vi "Read S-parameter Magnitude-Phase Pair.vi"(8 "error in (no error)":errorcluster, 10 "S-parameter Type (0: S11)":i32(ring) items=["S11", "S12", "S21", "S22"], 11 "VISA resource name":refnum<visa-resource-name>) -> (0 "error out":errorcluster, 1 "Current Phase":dbl, 2 "Current Magnitude":dbl, 3 "VISA resource name out":refnum<visa-resource-name>)   [LabVIEW 2014, in "Agilent U2000 Series.lvlib"]
doc: "Reads the current magnitude-phase pair values for the specified S-parameter type.\n\nNote: \nThis VI is only applicable for U2040 X-Series."
uses:
  Agilent U2000 Series.lvlib
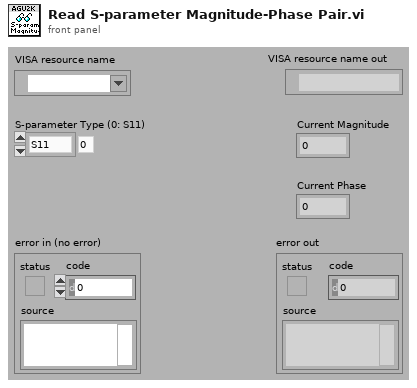
[diagram p1: front panel]
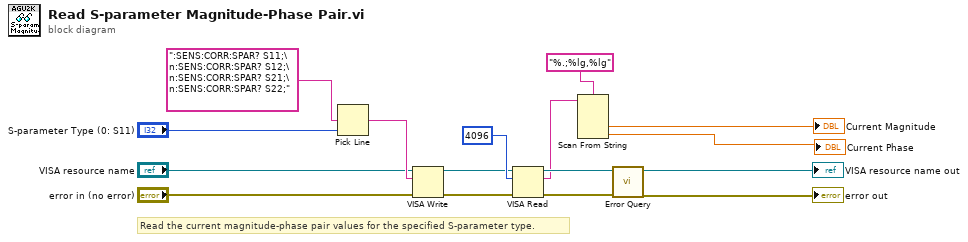
[diagram p0: block diagram]
diagram:
  # "Read the current magnitude-phase pair values for the specified S-parameter type."
  n1 = Pick Line(multi-line string=":SENS:CORR:SPAR? S11;\n:SENS:CORR:SPAR? S12;\n:SENS:CORR:SPAR? S21;\n:SENS:CORR:SPAR? S22;", line index="S-parameter Type (0: S11)") -> (output string=w14:string)  [unwired: 1 in]
  n2 = VISA Write(VISA resource name="VISA resource name", write buffer=w14, error in (no error)="error in (no error)") -> (VISA resource name out=w10:refnum<visa-resource-name>, error out=w9:errorcluster)  [unwired: 1 out]
  n3 = VISA Read(VISA resource name=w10, byte count=u32 4096, error in (no error)=w9) -> (VISA resource name out=w8:refnum<visa-resource-name>, read buffer=w4:string, error out=w7:errorcluster)  [unwired: 1 out]
  n4 = Scan From String(format string="%.;%lg,%lg", input string=w4) -> (output 1=→"Current Magnitude":dbl, output 2=→"Current Phase":dbl)  [unwired: 4 in, 3 out]
  n5 = call "Error Query.vi"("error in (no error)"=w7, "VISA resource name"=w8) -> ("error out"=→"error out":errorcluster, "VISA resource name out"=→"VISA resource name out":refnum<visa-resource-name>)  [unwired: 6 in, 2 out]
